vi "Write PreparePassInGamePlaysEnum.vi"(8 "error in (no error)":errorcluster, 10 "PreparePassInGamePlaysEnum":T1[](array[typedef])=[enum."NormalGame", enum."PreparePassInGame1"], 11 "Ally in":refnum<class "Ally.lvclass">) -> (0 "error out":errorcluster, 3 "Ally out":refnum<class "Ally.lvclass">)   [LabVIEW 2023, in "Ally.lvclass"]
uses:
  Ally.lvclass
  Team_class/OffensivePlay.ctl
  Ally.lvclass/Ally.ctl
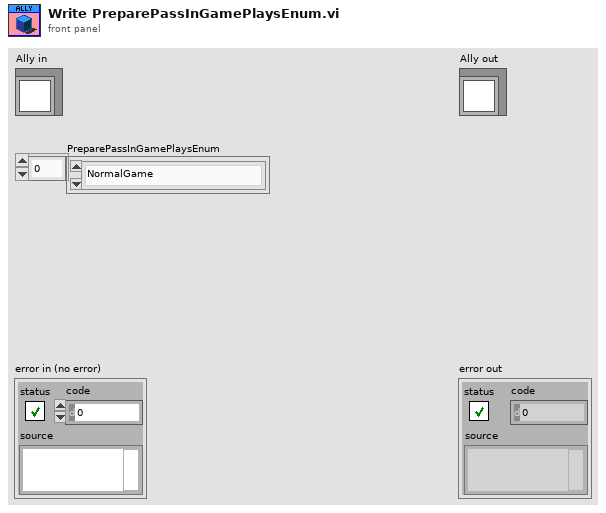
[diagram p1: front panel]
types:
  T1 = typedef "OffensivePlay.ctl" = enum16{"5RobotsPassGamePlay", "5PreparePassGame", "5RobotsKeeperGame", "KeeperPassToStriker", "5RobotsNormalGamePlay", "PrepareKeeperPass", "ACBPass", "ABCPass", "PrepareTriplePass", "TableWithStriker", "TableWith2ndStrikerPlay", "PrepareDoublePass", "PrepareRollToPass", "SimplePass", "PreparePass", "PassToStriker", "BallOutOfField", "PassTo2ndStriker", "StopOffensive", "Prepare Penalty Enemy", "EnemyPossessionAtEnemyField", "EnemyPossesionAtOurField", "TestPlay", "PreparePenaltyAlly", "KickPenaltyAlly", "PrepareKickoffAlly", "PrepareKickoffEnemy", "IndirectEnemy", "DirectEnemy", "PreparePassInGame1", "NormalGame", "DirectKick", "Pass", "Halt", "Timeout", "PassPlay", "PenaltyEnemy"}
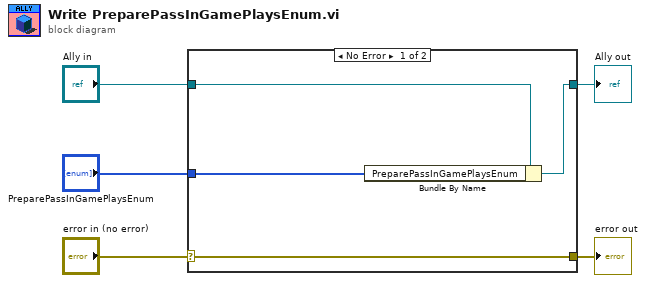
[diagram p0: block diagram]
diagram:
  n1 = case shown="No Error" "error in (no error)" {
    selector: "error in (no error)" -> [w9 w10]
    tunnel: [w9 w10] -> w4
    tunnel: [w7 w11] -> w2
    tunnel: "Ally in" -> [w8 w11]
    tunnel: "PreparePassInGamePlaysEnum" -> [w6 _]
    frame No Error {
      n2 = Bundle By Name(cluster=w8, "PreparePassInGamePlaysEnum"=w6) -> (w7:refnum<class "Ally.lvclass">)
    }
    frame Error {
    }
  }
  "error out" <- w4
  "Ally out" <- w2
